vi "_macro_Choreo_ReadAllTrajectories.vi"() -> ()   [LabVIEW 2019, in "ChoreoLib.lvlib"]
uses:
  ChoreoLib.lvlib
panel:
  out "Trajectories":string[](array[string])
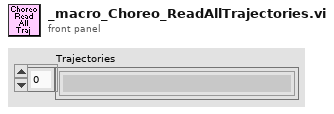
[diagram p1: front panel]
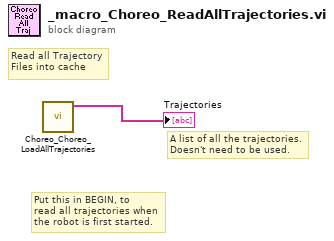
[diagram p0: block diagram]
diagram:
  # "Put this in BEGIN, to\nread all trajectories when\nthe robot is first started."
  # "A list of all the trajectories.\nDoesn't need to be used."
  # "Read all Trajectory\nFiles into cache"
  n1 = call "Choreo_Choreo_LoadAllTrajectories.vi"() -> ("Trajectories"=→"Trajectories":string[])  [unwired: 10 in, 1 out]
